vi "PS Control labactor.vi"() -> ()   [LabVIEW 2019]
uses:
  Users/Shared/NML Data Acquisition/Monovu/Monovu subvis/PS Status.ctl
  Stepper Controller/Serial Support VISA.llb/Serial Actions.ctl
  publisher action.ctl
  icicle.ctl
panel:
  in  "Tab Control":enum32{"Control", "Statistics"}(tab)
  out "Low":bool
  out "Total Remaining\nEnergy MW-hr":dbl(knob) scale=0.0..10.0
  out "Field [T]":dbl caption="Current [kA]" format="%.5f"
  in  "Setpoint [T]":dbl caption="(35.05) Max)" step=1e-05 format="%.5f"
  out "Field Display":cluster{dbl, dbl}(slide)={0.0, -0.0065359477124182705} scale=-35.046803202817955..35.046803202817955 scale format="%.1f"
  in  "Slew Rate [T/min]":dbl=0.001 caption="(10.850) Max)" min=0.001 max=50.0 step=0.01 format="%.3f"
  in  "stop":bool
  out "Status":T1
  out "Current [kA]":dbl format="%.5f"
  out "Current Display":cluster{dbl, dbl}(slide)={0.0, -0.0065359477124182705} scale=-38.8..38.8
  in  "FRTZ":bool
  in  "Pause":bool
  in  "Ramp":bool
  in  "Setpoint [kA]":dbl caption="(38.8) Max)" step=1e-05 format="%.5f"
  out "Cell":string
  in  "Slew Rate [A/s]":dbl=0.1 caption="(200.0) Max)" min=0.1 max=4000.0 step=10.0 format="%.1f"
  in  "Units":enum32{"tesla", "kAmps"}(radio) caption="tesla            kAmps"
  out "Power Level [MW]":dbl format="%.1g"
  in  "Reset Stats":bool
  out "Command Errors":i32
  out "% errors":dbl format="%.2f"
  out "Commands":string[](array[string])
  out "Errors":string[](array[string])
  out "Comm Rate [Hz]":dbl format="%.1f"
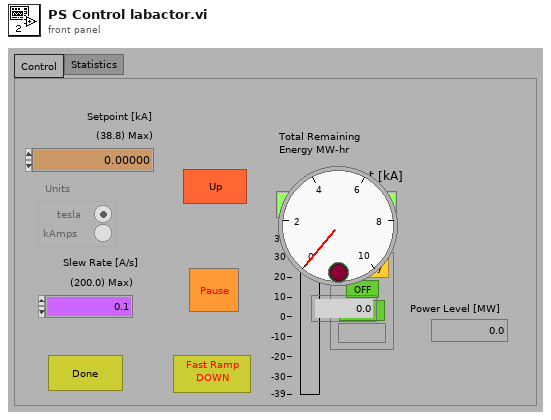
[diagram p1: front panel]
types:
  T1 = typedef "PS Status.ctl" = cluster{"PS On":bool, "PS Fault":bool, "Ramp Status":u16, "Cell Control":bool}
  T2 = typedef "Serial Actions.ctl" = enum16{"Init", "Break", "Clear Buffer", "Write", "Read", "N Bytes", "Lock", "Unlock", "Close"}
  T3 = cluster{"Minimum":dbl, "Maximum":dbl, "Increment":dbl}
  T4 = typedef "RMPS Magnet Config.ctl" = cluster{"#Coils":u32, "Coil Inductances":dbl[], "Maximum Coil Currents":dbl[], "Maximum Coil Voltage Deviation":dbl[], "Coil Coefficients":dbl[][], "Maximum Coil Temperatures":dbl[], " Pressure Range":dbl[], "Temp Coef":dbl[], "Offsets":dbl[], "Scale Factors":dbl[], "Cell Name":string}
  T5 = typedef "icicle.ctl" = cluster{"name":string, "units":string, "data":dbl}
  T6 = typedef "publisher action.ctl" = enum16{"set", "get", "init", "check"}
  T7 = enum8{"Enabled", "Disabled", "Disabled and Grayed Out"}
  T8 = cluster{bool, bool, "Ramp Status":u16, bool, bool, bool, bool}
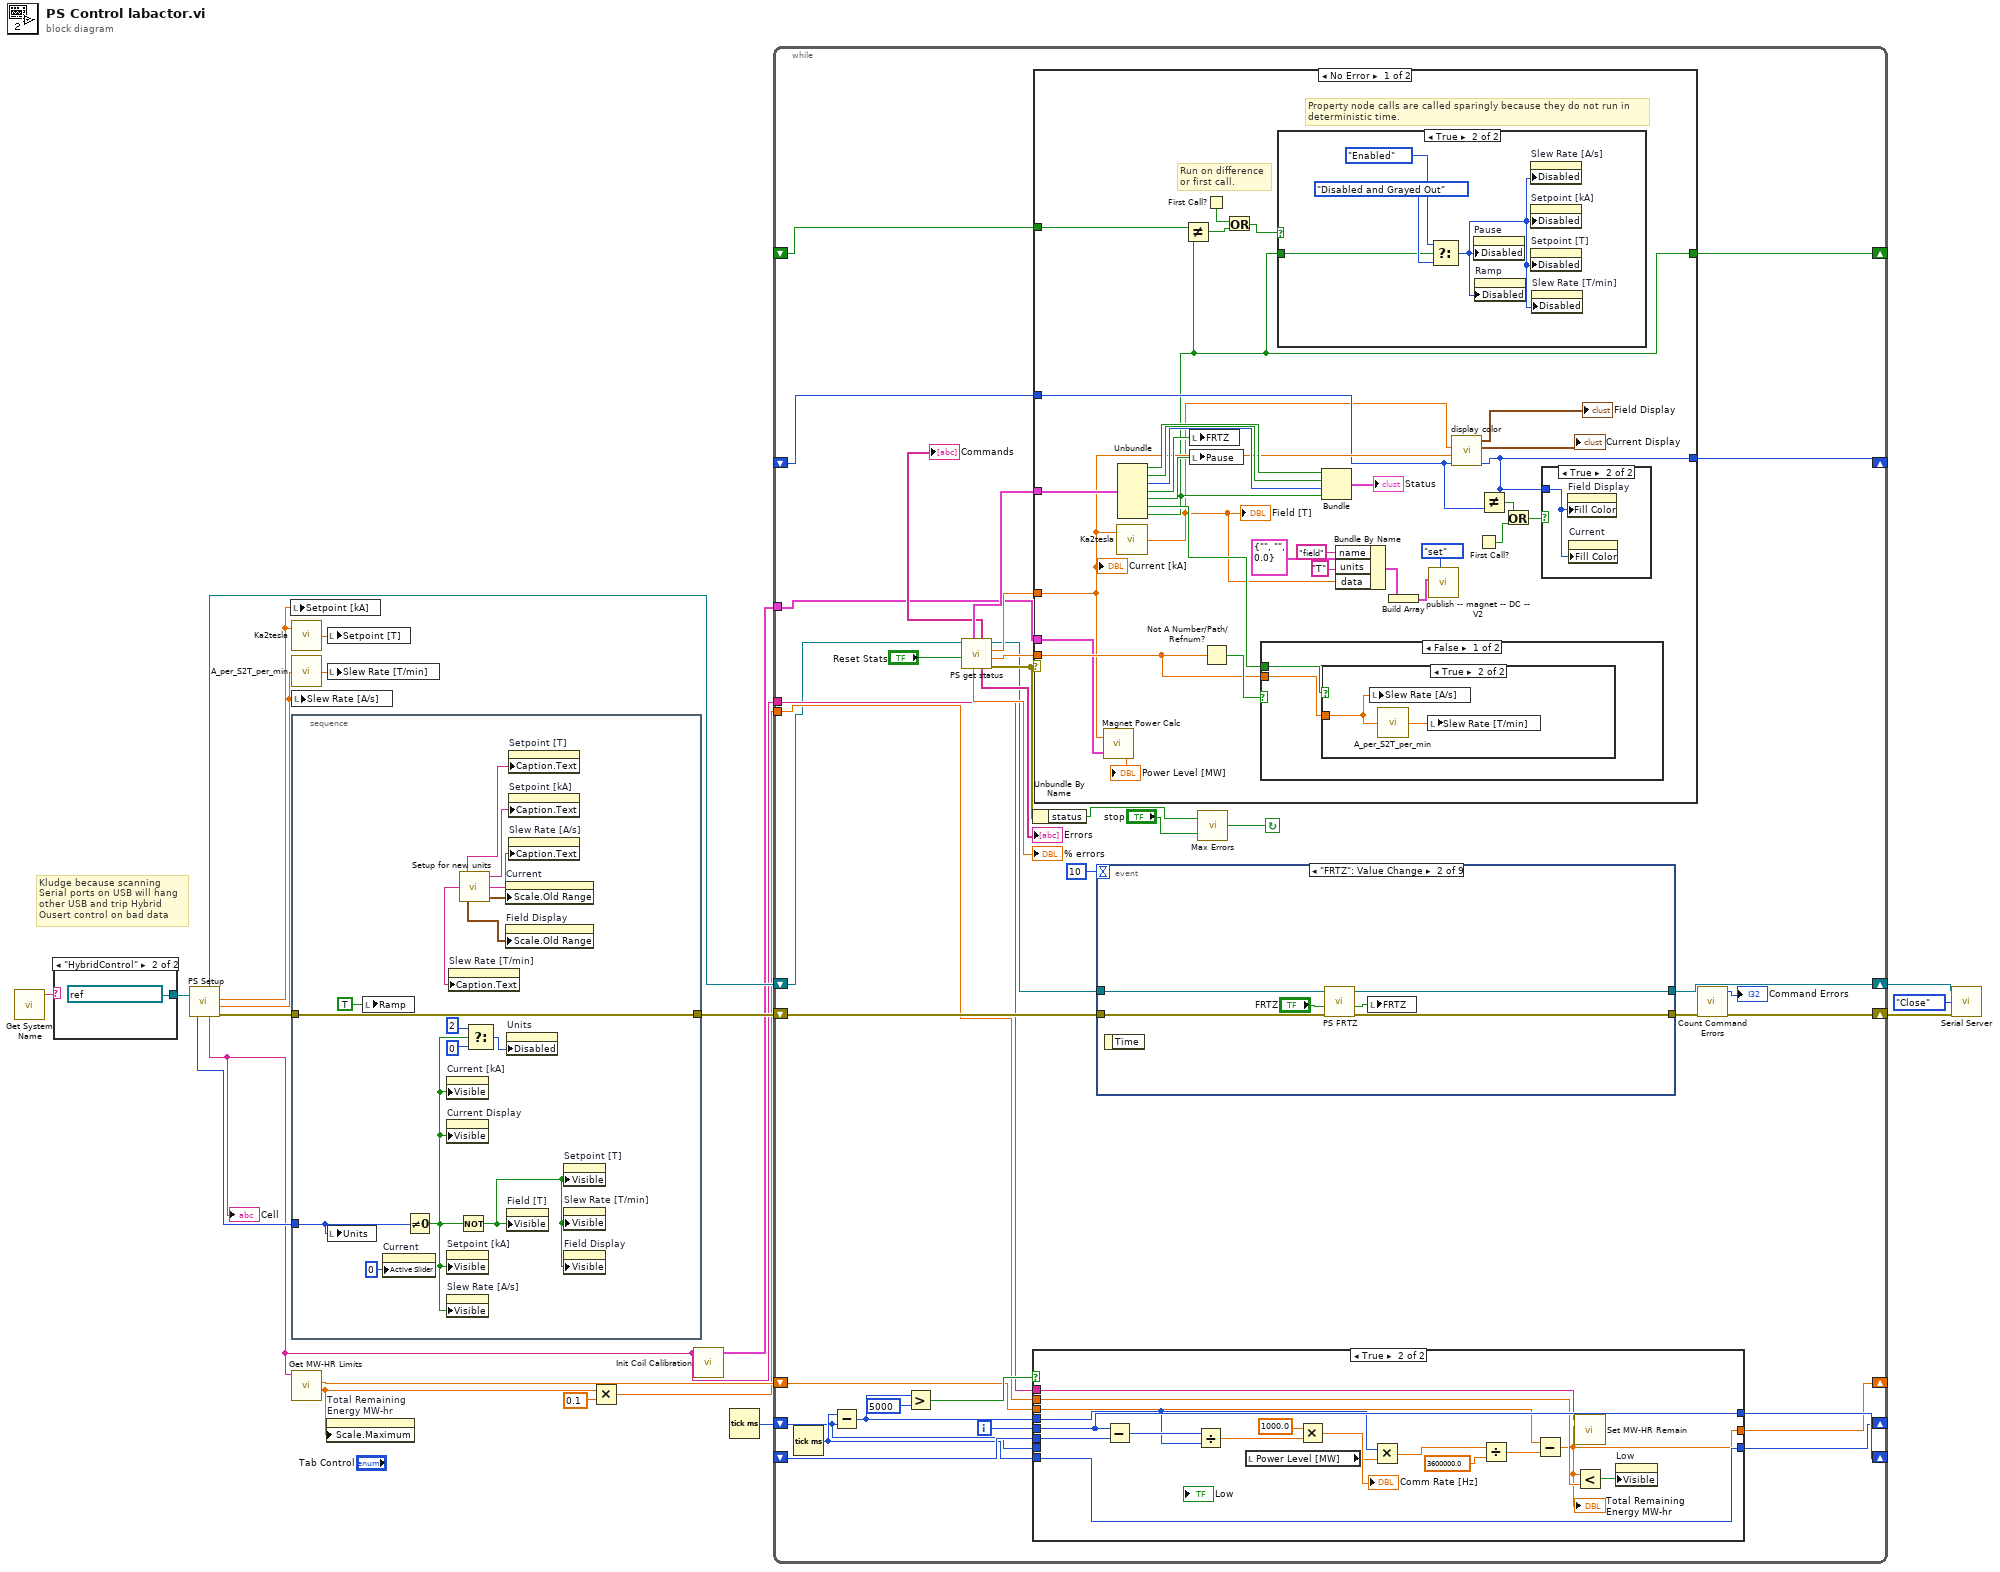
[diagram p0: block diagram]
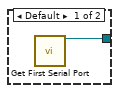
[diagram p2: hidden frame]
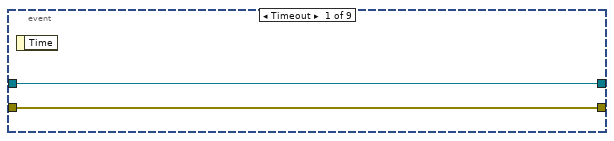
[diagram p4: hidden frame]
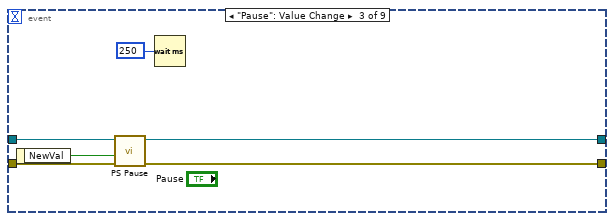
[diagram p5: hidden frame]
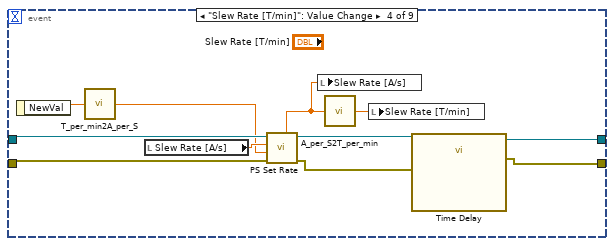
[diagram p6: hidden frame]
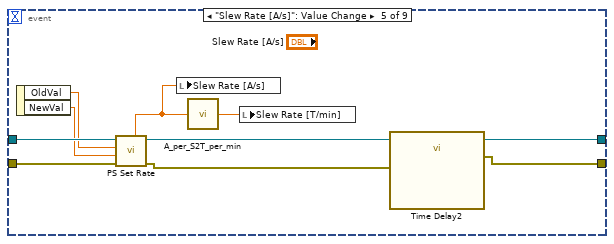
[diagram p7: hidden frame]
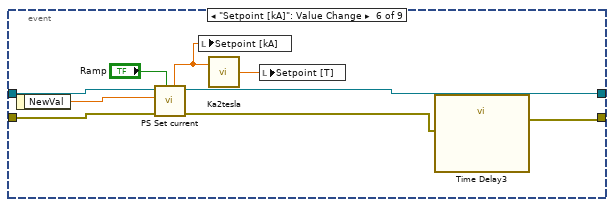
[diagram p8: hidden frame]
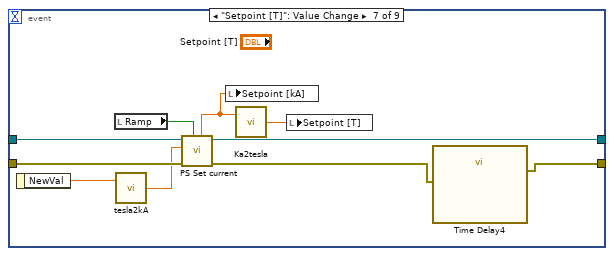
[diagram p9: hidden frame]
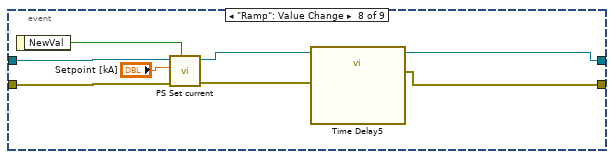
[diagram p10: hidden frame]
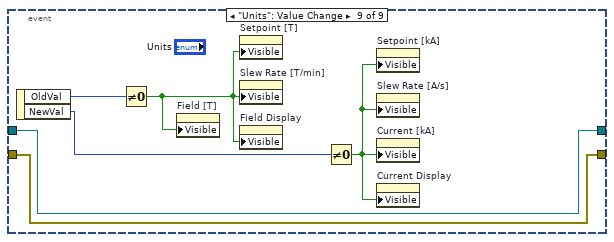
[diagram p11: hidden frame]
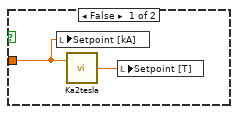
[diagram p14: hidden frame]
diagram:
  # "Kludge because scanning\nSerial ports on USB will hang\nother USB and trip Hybrid\nOusert control on bad data"
  n1 = call "Get System Name.vi"() -> ("System Name"=w2:string)  [unwired: 6 in, 1 out]
  n2 = case shown="\"HybridControl\"" w2 {
    tunnel: [w21 refnum<visa-resource-name> "Cell15Comm" ("PS Comm Port")] -> w1
    frame Default {
      n3 = call "Get First Serial Port.vi"() -> ("PS Comm Port"=w21:refnum<visa-resource-name>)  [unwired: 14 in, 1 out]
    }
    frame "HybridControl" {
    }
  }
  n4 = call "PS Setup.vi"("PS Communication Port"=w1) -> ("Units"=w20:enum32{"tesla", "kAmps"}, "dup VISA Resource Name"=w17:refnum<visa-resource-name>, "Cell"=w4:string, "Setpoint"=w15:dbl, "Slew Rate"=w13:dbl, "error out"=w11:errorcluster)  [unwired: 1 in]
  "Cell" <- w4
  n5 = local write "Setpoint [kA]"(w15) -> ()
  n6 = call "Ka2tesla.vi"("Magnet Current [kA]"=w15) -> ("Field"=w16:dbl)  [unwired: 1 in]
  n7 = call "A_per_S2T_per_min.vi"("A/sec"=w13) -> ("T/min"=w14:dbl)
  n8 = local write "Slew Rate [A/s]"(w13) -> ()
  n9 = stacked-sequence {
    tunnel: w20 -> [w24]
    tunnel: [w27] -> w12
    tunnel: w11 -> [w27]
    frame #0 {
      n10 = local write "Units"(w24) -> ()
      n11 = local write "Ramp"(TRUE) -> ()
      n12 = property on="Current" class="Slide (strict)"("Active Slider"=0 ("Write Attribute")) -> ()  [unwired: 2 in, 2 out]
      n13 = Not Equal To 0?(x=w24) -> (x != 0?=w23:bool)
      n14 = property on="Current [kA]" class="DigNum (strict)"("Visible"=w23) -> ()  [unwired: 2 in, 2 out]
      n15 = property on="Current Display" class="Slide (strict)"("Visible"=w23) -> ()  [unwired: 2 in, 2 out]
      n16 = property on="Setpoint [kA]" class="DigNum (strict)"("Visible"=w23) -> ()  [unwired: 2 in, 2 out]
      n17 = property on="Slew Rate [A/s]" class="DigNum (strict)"("Visible"=w23) -> ()  [unwired: 2 in, 2 out]
      n18 = Not(x=w23) -> (.not. x?=w25:bool)
      n19 = call "Setup for new units.vi"() -> ("Current Range"=w33:T3, "Current Slew Rate Caption"=w32:string, "Current Setpoint Caption"=w31:string, "Field Range"=w30:T3, "Field Slew Rate Caption"=w29:string, "Field Setpoint Caption"=w28:string)
      n20 = property on="Slew Rate [T/min]" class="DigNum (strict)"("Caption.Text"=w29) -> ()  [unwired: 2 in, 2 out]
      n21 = Select(t=u8 2, s=w23, f=u8 0) -> (s? t:f=w35:u8)
      n22 = property on="Current" class="Slide (strict)"("Scale.Old Range"=w33) -> ()  [unwired: 2 in, 2 out]
      n23 = property on="Field Display" class="Slide (strict)"("Scale.Old Range"=w30) -> ()  [unwired: 2 in, 2 out]
      n24 = property on="Units" class="RadioBtnsControl (strict)"("Disabled"=w35) -> ()  [unwired: 2 in, 2 out]
      n25 = property on="Field [T]" class="DigNum (strict)"("Visible"=w25) -> ()  [unwired: 2 in, 2 out]
      n26 = property on="Setpoint [T]" class="DigNum (strict)"("Caption.Text"=w28) -> ()  [unwired: 2 in, 2 out]
      n27 = property on="Setpoint [kA]" class="DigNum (strict)"("Caption.Text"=w31) -> ()  [unwired: 2 in, 2 out]
      n28 = property on="Slew Rate [A/s]" class="DigNum (strict)"("Caption.Text"=w32) -> ()  [unwired: 2 in, 2 out]
      n29 = property on="Setpoint [T]" class="DigNum (strict)"("Visible"=w25) -> ()  [unwired: 2 in, 2 out]
      n30 = property on="Slew Rate [T/min]" class="DigNum (strict)"("Visible"=w25) -> ()  [unwired: 2 in, 2 out]
      n31 = property on="Field Display" class="Slide (strict)"("Visible"=w25) -> ()  [unwired: 2 in, 2 out]
    }
  }
  n32 = call "Get MW-HR Limits.vi"("Cell"=w4) -> ("Max MW-HR"=w3:dbl, "MW-HR Remain"=w7:dbl)  [unwired: 8 in, 1 out]
  n33 = property on="Total Remaining\nEnergy MW-hr" class="Knob (strict)"("Scale.Maximum"=w3) -> ()  [unwired: 2 in, 2 out]
  n34 = local write "Setpoint [T]"(w16) -> ()
  n35 = local write "Slew Rate [T/min]"(w14) -> ()
  n36 = Multiply(x=w3, y=0.1) -> (x*y=w5:dbl)
  n37 = call "Init Coil Calibration.vi"("Magnet ID"=w4) -> ("Magnet Configuration Data"=w8:T4)  [unwired: 2 in, 4 out]
  n38 = Tick Count (ms)() -> (millisecond timer value=w9:u32)
  n39 = while {
    shift-right: [w44] -> w10
    shift-left: w12 -> [w55]
    shift-right: [w58] -> _
    shift-left: w9 -> [w59]
    shift-right: [w61] -> _
    shift-left: _ -> [w62]
    tunnel: w8 -> [w53]
    shift-right: [w51] -> _
    shift-left: w7 -> [w52]
    tunnel: w5 -> [w50]
    tunnel: w4 -> [w49]
    shift-right: [w47] -> w18
    shift-left: w17 -> [w48]
    shift-right: [w41] -> _
    shift-left: _ -> [w40]
    shift-right: [w39] -> _
    shift-left: _ -> [w38]
    i -> [w63]
    stop <- w72 continue-if-true
    n40 = Tick Count (ms)() -> (millisecond timer value=w60:u32)
    n41 = Subtract(x=w60, y=w59) -> (x-y=w64:u32)
    n42 = Greater?(x=w64, y=u32 5000) -> (0:w65:bool)
    n43 = call "PS get status.vi"("Reset"="Reset Stats", "VISA Resource Name"=w48) -> ("error out"=w67:errorcluster, "Setpoint"=w73:dbl, "Current"=w69:dbl, "dup VISA Resource Name"=w46:refnum<visa-resource-name>, "Errors Out"=→"Errors":string[], "Commands Out"=→"Commands":string[], "% errors"=→"% errors":dbl, "Status"=w74:T8)  [unwired: 2 in]
    n44 = Unbundle By Name(w67) -> ("status"=w68:bool)
    n45 = case shown="True" w65 {
      tunnel: w64 -> [_ w86]
      tunnel: w63 -> [_ w93]
      tunnel: w62 -> [w76 w94]
      tunnel: [w76 w93] -> w61
      tunnel: w60 -> [_ w88]
      tunnel: w59 -> [w77 _]
      tunnel: [w77 w88] -> w58
      tunnel: w52 -> [w75 w82]
      tunnel: [w75 w79] -> w51
      tunnel: w50 -> [_ w80]
      tunnel: w49 -> [_ w78]
      frame False {
      }
      frame True {
        n46 = Subtract(x=w93, y=w94) -> (x-y=w92:i32)
        n47 = Divide(x=w92, y=w86) -> (x/y=w91:dbl)
        n48 = local read "Power Level [MW]"() -> (w87:dbl)
        n49 = Multiply(x=1000.0, y=w91) -> (x*y=→"Comm Rate [Hz]":dbl)
        n50 = Multiply(x=w86, y=w87) -> (x*y=w85:dbl)
        n51 = Divide(x=w85, y=3600000.0) -> (x/y=w83:dbl)
        n52 = Subtract(x=w82, y=w83) -> (x-y=w79:dbl)
        "Total Remaining\nEnergy MW-hr" <- w79
        n53 = call "Set MW-HR Remain.vi"("MW-HR Remain"=w79, "Cell"=w78) -> ()  [unwired: 9 in, 1 out]
        n54 = Less?(x=w79, y=w80) -> (x < y?=w81:bool)
        n55 = property on="Low" class="Bool (strict)"("Visible"=w81) -> ()  [unwired: 2 in, 2 out]
      }
    }
    n56 = case shown="No Error" w67 {
      tunnel: w74 -> [w187 _]
      tunnel: w69 -> [w179 _]
      tunnel: w73 -> [w183 _]
      tunnel: w53 -> [w180 _]
      tunnel: [w167 w203] -> w41
      tunnel: w40 -> [w176 w203]
      tunnel: [w174 w204] -> w39
      tunnel: w38 -> [w175 w204]
      frame No Error {
        # "Property node calls are called sparingly because they do not run in\ndeterministic time."
        # "Run on difference\nor first call."
        n57 = call "Magnet Power Calc.vi"("Current"=w179, "Magnet Configuration Data"=w180) -> ("Power"=→"Power Level [MW]":dbl)  [unwired: 3 out]
        n58 = call "Ka2tesla.vi"("Magnet Current [kA]"=w179) -> ("Field"=w163:dbl)  [unwired: 1 in]
        "Field [T]" <- w163
        n59 = Unbundle(w187) -> (w188:bool, w190:bool, "Ramp Status"=w191:u16, w182:bool, w181:bool, w184:bool, w174:bool)
        n60 = Not Equal?(x=w175, y=w174) -> (x != y?=w172:bool)
        n61 = local write "FRTZ"(w182) -> ()
        n62 = local write "Pause"(w181) -> ()
        n63 = First Call?() -> (First Call?: T/F=w173:bool)
        n64 = Not A Number/Path/Refnum?(number/path/refnum=w183) -> (NaN/Path/Refnum?=w185:bool)
        n65 = Or(x=w173, y=w172) -> (x .or. y?=w171:bool)
        n66 = case shown="False" w185 {
          tunnel: w184 -> [w198 _]
          tunnel: w183 -> [w197 _]
          frame False {
            n67 = case shown="True" w198 {
              tunnel: w197 -> [w199 w201]
              frame False {
                n68 = local write "Setpoint [kA]"(w199) -> ()
                n69 = call "Ka2tesla.vi"("Magnet Current [kA]"=w199) -> ("Field"=w200:dbl)  [unwired: 1 in]
                n70 = local write "Setpoint [T]"(w200) -> ()
              }
              frame True {
                n71 = local write "Slew Rate [A/s]"(w201) -> ()
                n72 = call "A_per_S2T_per_min.vi"("A/sec"=w201) -> ("T/min"=w202:dbl)
                n73 = local write "Slew Rate [T/min]"(w202) -> ()
              }
            }
          }
          frame True {
          }
        }
        n74 = case shown="True" w171 {
          tunnel: w174 -> [_ w192]
          frame False {
          }
          frame True {
            n75 = Select(t=T7."Enabled" ("Disabled"), s=w192, f=T7."Disabled and Grayed Out" ("Disabled")) -> (s? t:f=w195:T7)
            n76 = property on="Pause" class="Bool (strict)"("Disabled"=w195) -> ()  [unwired: 2 in, 2 out]
            n77 = property on="Ramp" class="Bool (strict)"("Disabled"=w195) -> ()  [unwired: 2 in, 2 out]
            n78 = property on="Slew Rate [A/s]" class="DigNum (strict)"("Disabled"=w195) -> ()  [unwired: 2 in, 2 out]
            n79 = property on="Setpoint [kA]" class="DigNum (strict)"("Disabled"=w195) -> ()  [unwired: 2 in, 2 out]
            n80 = property on="Setpoint [T]" class="DigNum (strict)"("Disabled"=w195) -> ()  [unwired: 2 in, 2 out]
            n81 = property on="Slew Rate [T/min]" class="DigNum (strict)"("Disabled"=w195) -> ()  [unwired: 2 in, 2 out]
          }
        }
        n82 = Bundle(w188, w190, "Ramp Status"=w191, w174) -> (→"Status":cluster{bool, bool, "Ramp Status":u16, bool})  [unwired: 1 in]
        n83 = Bundle By Name(cluster=T5 {"name"="", "units"="", "data"=0.0} ("icicle"), "name"="field", "units"="T", "data"=w163) -> (w161:T5)
        n84 = Build Array(w161) -> (w160:T5[])
        n85 = call "publish -- magnet -- DC -- V2.vi"("publisher action"=publisher_action."set", "Array"=w160) -> ()  [unwired: 9 in, 1 out]
        n86 = call "display color.vi"("Existing fill color"=w176, "Current"=w179, "Field"=w163) -> ("Fill Color"=w167:u32, "Current"=→"Current Display":cluster{dbl, dbl}, "Field"=→"Field Display":cluster{dbl, dbl})  [unwired: 4 in]
        n87 = First Call?() -> (First Call?: T/F=w169:bool)
        n88 = Not Equal?(x=w167, y=w176) -> (x != y?=w170:bool)
        n89 = Or(x=w170, y=w169) -> (x .or. y?=w168:bool)
        n90 = case shown="True" w168 {
          tunnel: w167 -> [_ w196]
          frame False {
          }
          frame True {
            n91 = property on="Field Display" class="Slide (strict)"("Fill Color"=w196) -> ()  [unwired: 2 in, 2 out]
            n92 = property on="Current" class="Slide (strict)"("Fill Color"=w196) -> ()  [unwired: 2 in, 2 out]
          }
        }
        "Current [kA]" <- w179
      }
      frame Error {
      }
    }
    n93 = event shown="[1] \"FRTZ\": Value Change" {
      selector: _ -> [_ _ _ _ _ _ _ _ _]
      dyn-events: _ -> [_ _ _ _ _ _ _ _ _]
      timeout: 10 -> [_ _ _ _ _ _ _ _ _]
      tunnel: w55 -> [w96 w102 w105 w117 w126 w135 w145 w152 w157]
      tunnel: [w96 w101 w104 w109 w119 w128 w137 w148 w157] -> w45
      tunnel: w46 -> [w95 w100 w106 w118 w127 w136 w146 w153 w154]
      tunnel: [w95 w97 w103 w111 w121 w130 w139 w149 w154] -> w47
      event Timeout {
        n94 = event-data() -> ()  [unwired: 1 in, 1 out]
      }
      event "FRTZ": Value Change {
        n95 = event-data() -> ()  [unwired: 1 in, 1 out]
        n96 = call "PS FRTZ.vi"("error In"=w102, "FRTZ"="FRTZ", "VISA Resource Name"=w100) -> ("error out"=w101:errorcluster, "FRTZ Out"=w98:bool, "dup VISA Resource Name"=w97:refnum<visa-resource-name>)  [unwired: 2 in]
        n97 = local write "FRTZ"(w98) -> ()
      }
      event "Pause": Value Change {
        n98 = event-data() -> ("NewVal"=w108:bool)  [unwired: 1 in]
        n99 = call "PS Pause.vi"("error In"=w105, "Pause"=w108, "VISA Resource Name"=w106) -> ("error out"=w104:errorcluster, "dup VISA Resource Name"=w103:refnum<visa-resource-name>)  [unwired: 3 in]
        n100 = Wait (ms)(milliseconds to wait=u32 250) -> ()  [unwired: 1 out]
      }
      event "Slew Rate [T/min]": Value Change {
        n101 = event-data() -> ("NewVal"=w114:dbl)  [unwired: 1 in]
        n102 = call "T_per_min2A_per_S.vi"("T/min"=w114) -> ("A/sec"=w115:dbl)
        n103 = local read "Slew Rate [A/s]"() -> (w116:dbl)
        n104 = call "PS Set Rate.vi"("VISA Resource Name"=w118, "Old Slew Rate"=w116, "Slew Rate [A/S]"=w115, "error In"=w117) -> ("Slew Rate Out [A/S]"=w113:dbl, "dup VISA Resource Name"=w111:refnum<visa-resource-name>, "error Out"=w110:errorcluster)  [unwired: 1 in, 1 out]
        n105 = local write "Slew Rate [A/s]"(w113) -> ()
        n106 = call "A_per_S2T_per_min.vi"("A/sec"=w113) -> ("T/min"=w112:dbl)
        n107 = local write "Slew Rate [T/min]"(w112) -> ()
        n108 = call "Time Delay"("error in (no error)"=w110) -> ("error out"=w109:errorcluster)  [unwired: 10 in]
      }
      event "Slew Rate [A/s]": Value Change {
        n109 = event-data() -> ("OldVal"=w125:dbl, "NewVal"=w124:dbl)  [unwired: 1 in]
        n110 = call "PS Set Rate.vi"("VISA Resource Name"=w127, "Old Slew Rate"=w125, "Slew Rate [A/S]"=w124, "error In"=w126) -> ("Slew Rate Out [A/S]"=w123:dbl, "dup VISA Resource Name"=w121:refnum<visa-resource-name>, "error Out"=w120:errorcluster)  [unwired: 1 in, 1 out]
        n111 = local write "Slew Rate [A/s]"(w123) -> ()
        n112 = call "A_per_S2T_per_min.vi"("A/sec"=w123) -> ("T/min"=w122:dbl)
        n113 = local write "Slew Rate [T/min]"(w122) -> ()
        n114 = call "Time Delay2"("error in (no error)"=w120) -> ("error out"=w119:errorcluster)  [unwired: 10 in]
      }
      event "Setpoint [kA]": Value Change {
        n115 = event-data() -> ("NewVal"=w132:dbl)  [unwired: 1 in]
        n116 = call "PS Set current.vi"("Ramp"="Ramp", "error In"=w135, "SetPoint"=w132, "VISA Resource Name"=w136) -> ("error out"=w129:errorcluster, "dup VISA Resource Name"=w130:refnum<visa-resource-name>, "SetPoint Out"=w133:dbl)  [unwired: 3 in, 1 out]
        n117 = local write "Setpoint [kA]"(w133) -> ()
        n118 = call "Ka2tesla.vi"("Magnet Current [kA]"=w133) -> ("Field"=w134:dbl)  [unwired: 1 in]
        n119 = local write "Setpoint [T]"(w134) -> ()
        n120 = call "Time Delay3"("error in (no error)"=w129) -> ("error out"=w128:errorcluster)  [unwired: 10 in]
      }
      event "Setpoint [T]": Value Change {
        n121 = event-data() -> ("NewVal"=w142:dbl)  [unwired: 1 in]
        n122 = local read "Ramp"() -> (w140:bool)
        n123 = call "tesla2kA.vi"("Magnet Filed [T]"=w142) -> ("Current [kA]"=w141:dbl)  [unwired: 1 in]
        n124 = call "PS Set current.vi"("Ramp"=w140, "error In"=w145, "SetPoint"=w141, "VISA Resource Name"=w146) -> ("error out"=w138:errorcluster, "dup VISA Resource Name"=w139:refnum<visa-resource-name>, "SetPoint Out"=w143:dbl)  [unwired: 3 in, 1 out]
        n125 = local write "Setpoint [kA]"(w143) -> ()
        n126 = call "Ka2tesla.vi"("Magnet Current [kA]"=w143) -> ("Field"=w144:dbl)  [unwired: 1 in]
        n127 = local write "Setpoint [T]"(w144) -> ()
        n128 = call "Time Delay4"("error in (no error)"=w138) -> ("error out"=w137:errorcluster)  [unwired: 10 in]
      }
      event "Ramp": Value Change {
        n129 = event-data() -> ("NewVal"=w150:bool)  [unwired: 1 in]
        n130 = call "PS Set current.vi"("Ramp"=w150, "error In"=w152, "SetPoint"="Setpoint [kA]", "VISA Resource Name"=w153) -> ("error out"=w147:errorcluster, "dup VISA Resource Name"=w149:refnum<visa-resource-name>)  [unwired: 3 in, 2 out]
        n131 = call "Time Delay5"("error in (no error)"=w147) -> ("error out"=w148:errorcluster)  [unwired: 10 in]
      }
      event "Units": Value Change {
        n132 = event-data() -> ("OldVal"=w158:enum32{"tesla", "kAmps"}, "NewVal"=w159:enum32{"tesla", "kAmps"})  [unwired: 1 in]
        n133 = Not Equal To 0?(x=w158) -> (x != 0?=w156:bool)
        n134 = property on="Field [T]" class="DigNum (strict)"("Visible"=w156) -> ()  [unwired: 2 in, 2 out]
        n135 = property on="Setpoint [T]" class="DigNum (strict)"("Visible"=w156) -> ()  [unwired: 2 in, 2 out]
        n136 = property on="Slew Rate [T/min]" class="DigNum (strict)"("Visible"=w156) -> ()  [unwired: 2 in, 2 out]
        n137 = property on="Field Display" class="Slide (strict)"("Visible"=w156) -> ()  [unwired: 2 in, 2 out]
        n138 = Not Equal To 0?(x=w159) -> (x != 0?=w155:bool)
        n139 = property on="Setpoint [kA]" class="DigNum (strict)"("Visible"=w155) -> ()  [unwired: 2 in, 2 out]
        n140 = property on="Slew Rate [A/s]" class="DigNum (strict)"("Visible"=w155) -> ()  [unwired: 2 in, 2 out]
        n141 = property on="Current [kA]" class="DigNum (strict)"("Visible"=w155) -> ()  [unwired: 2 in, 2 out]
        n142 = property on="Current Display" class="Slide (strict)"("Visible"=w155) -> ()  [unwired: 2 in, 2 out]
      }
    }
    n143 = call "Max Errors.vi"("stop"="stop", "error"=w68) -> ("Cont?"=w72:bool)
    n144 = call "Count Command Errors.vi"("Error In"=w45) -> ("Error Out"=w44:errorcluster, "Command Errors"=→"Command Errors":i32)  [unwired: 9 in]
  }
  n145 = call "Serial Server.vi"("VISA Resource Name"=w18, "Action"=Serial_Actions."Close", "error in (no error)"=w10) -> ()  [unwired: 8 in, 5 out]
